vi "Broadcast Debug Data.vi"(8 "error in (no error)":errorcluster, 10 "Debug Data Cluster":T1, 11 "Debug Message Receiver in":refnum<class "Debug Message Receiver.lvclass">) -> (0 "error out":errorcluster, 3 "Debug Message Receiver out":refnum<class "Debug Message Receiver.lvclass">)   [LabVIEW 2020, in "Debug Message Receiver.lvclass"]
uses:
  Debug Message Receiver.lvclass
  Debug Message Receiver.lvclass/Debug Message Receiver.ctl
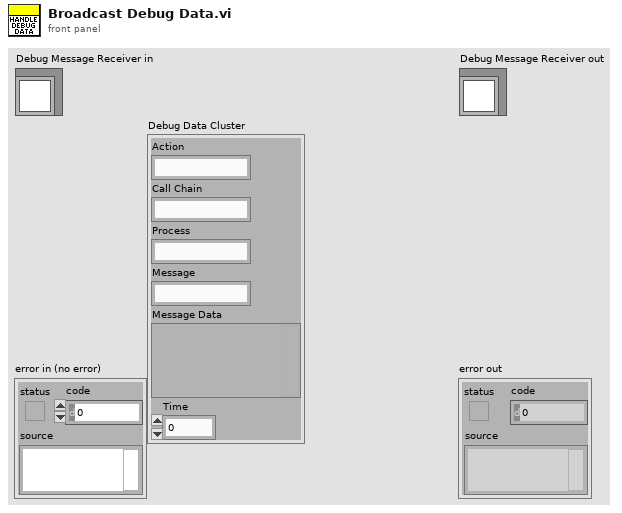
[diagram p1: front panel]
types:
  T1 = cluster{"Action":string, "Call Chain":string, "Process":string, "Message":string, "Message Data":variant, "Time":u32}
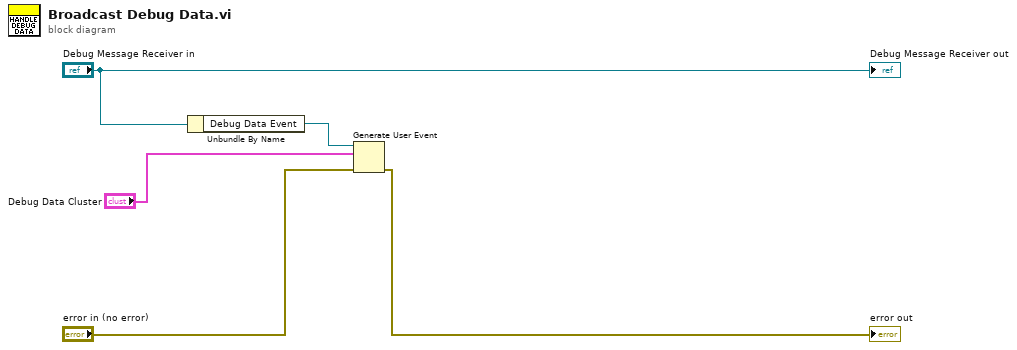
[diagram p0: block diagram]
diagram:
  n1 = Unbundle By Name("Debug Message Receiver in") -> ("Debug Data Event"=w5:refnum<user-event>)
  n2 = Generate User Event(user event=w5, event data cluster="Debug Data Cluster", error in="error in (no error)") -> (error out=→"error out":errorcluster)  [unwired: 1 in, 1 out]
  "Debug Message Receiver out" <- "Debug Message Receiver in"
